vi "Initialize.vi"(11 "Brick Wall in":refnum<class "Brick Wall.lvclass">) -> (3 "Brick Wall out":refnum<class "Brick Wall.lvclass">)   [LabVIEW 2015, in "Brick Wall.lvclass"]
uses:
  Brick Wall.lvclass
  Brick Wall Type.ctl
  Type Defs/Direction Enum.ctl
  SpawnLines.ctl
  Brick Wall.lvclass/Brick Wall.ctl
  Type Defs/SB Type Defs.lvlib
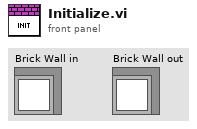
[diagram p1: front panel]
types:
  T1 = typedef "Brick Wall.lvclass/SpawnLines.ctl" = cluster{"NSpawn":i32, "ESpawn":i32, "SSpawn":i32, "WSpawn":i32}
  T2 = typedef "SB Type Defs.lvlib/Direction Enum.ctl" = enum16{"NW", "N", "NE", "E", "SE", "S", "SW", "W"}
  T3 = typedef "Brick Wall.lvclass/Brick Wall Type.ctl" = enum16{"Row Starter", "Mover", "Starter", "Spawner", "Mason", "Wall"}
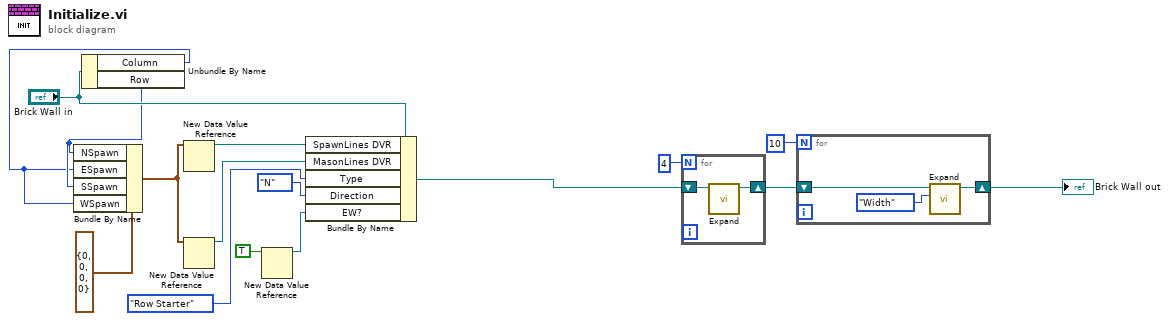
[diagram p0: block diagram]
diagram:
  n1 = Unbundle By Name("Brick Wall in") -> ("Column"=w2:i32, "Row"=w3:i32)
  n2 = Bundle By Name(cluster=T1 {"NSpawn"=0, "ESpawn"=0, "SSpawn"=0, "WSpawn"=0} ("WallLines"), "NSpawn"=w3, "ESpawn"=w2, "SSpawn"=w3, "WSpawn"=w2) -> (w1:T1)
  n3 = New Data Value Reference(data value=w1) -> (data value reference=w13:refnum<data-value>)  [unwired: 1 in, 1 out]
  n4 = New Data Value Reference(data value=w1) -> (data value reference=w8:refnum<data-value>)  [unwired: 1 in, 1 out]
  n5 = New Data Value Reference(data value=TRUE) -> (data value reference=w16:refnum<data-value>)  [unwired: 1 in, 1 out]
  n6 = Bundle By Name(cluster="Brick Wall in", "SpawnLines DVR"=w13, "MasonLines DVR"=w8, "Type"=Brick_Wall_Type."Row Starter" ("Player. Type"), "Direction"=Direction_Enum."N" ("Player.Direction"), "EW?"=w16) -> (w7:refnum<class "Brick Wall.lvclass">)
  n7 = for {
    N: 4 -> [_]
    shift-right: [w17] -> w5
    shift-left: w7 -> [w18]
    n8 = call-dynamic "Expand.vi"("Brick Wall in"=w18) -> ("Brick Wall out"=w17:refnum<class "Brick Wall.lvclass">)  [unwired: 9 in, 1 out]
  }
  n9 = for {
    N: 10 -> [_]
    shift-right: [w20] -> w11
    shift-left: w5 -> [w21]
    n10 = call-dynamic "Expand.vi"("Expand Direction"=enum16{"Height", "Width", "Both"}."Width", "Brick Wall in"=w21) -> ("Brick Wall out"=w20:refnum<class "Brick Wall.lvclass">)  [unwired: 8 in, 1 out]
  }
  "Brick Wall out" <- w11
